vi "Read myNum.vi"(8 "error in (no error)":errorcluster, 11 "Class3 in":refnum<class "Class3.lvclass">) -> (0 "error out":errorcluster, 2 "myNum":dbl, 3 "Class3 out":refnum<class "Class3.lvclass">)   [LabVIEW 2020, in "Class3.lvclass"]
doc: "GCraftsman JSON Object Serialization Toolkit\nwww.GCraftsman.com\nCopyright (c) 2017, GCraftsman"
uses:
  Class3.lvclass
  Class3.lvclass/Class3.ctl
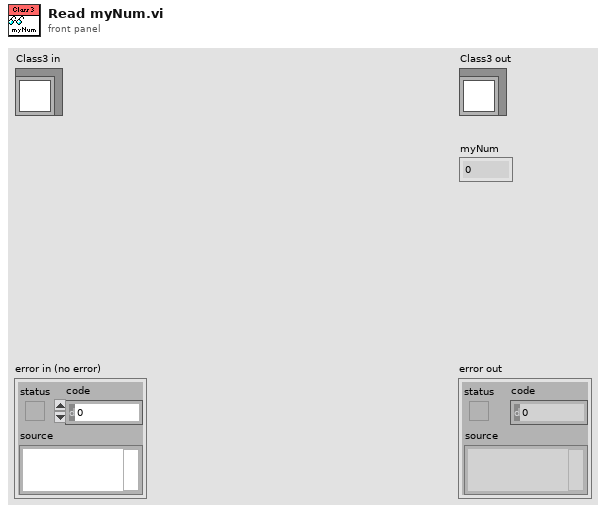
[diagram p1: front panel]
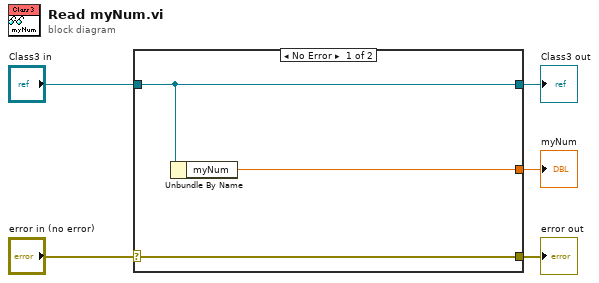
[diagram p0: block diagram]
diagram:
  n1 = case shown="No Error" "error in (no error)" {
    selector: "error in (no error)" -> [w8 w9]
    tunnel: [w8 w9] -> w4
    tunnel: [w7 w10] -> w2
    tunnel: "Class3 in" -> [w7 w10]
    tunnel: [w6 _] -> w1
    frame No Error {
      n2 = Unbundle By Name(w7) -> ("myNum"=w6:dbl)
    }
    frame Error {
    }
  }
  "error out" <- w4
  "Class3 out" <- w2
  "myNum" <- w1
